vi "Launch SM DI Threads.vi"(8 "error in (no error)":errorcluster, 10 "DAQ Process AppData":T1, 11 "DAQ in":refnum<class "DAQ.lvclass">) -> (0 "error out":errorcluster, 3 "DAQ out":refnum<class "DAQ.lvclass">)   [LabVIEW 2017, in "DAQ.lvclass"]
doc: "Developed by Kevin Thompson\nkevin@thompsonengineering.net\n\nCopyright 2018-2020\nThompson Engineering, LLC"
uses:
  DAQ.lvclass
  Process_DAQ SM AppData--cluster.ctl
  DataTypes/TD DAQ Settings--cluster.ctl
  DataTypes/TD DI Instrument Settings--cluster.ctl
  DataTypes/TD AI Instrument Settings--cluster.ctl
  DataTypes/TD AI InstSettings--cluster.ctl
  TD SimAI Ranges--cluster.ctl
  <vilib>/TELLC/Dynamic CVT API/TD Dynamic CVT DVR--ref.ctl
  DAQ.lvclass/DAQ.ctl
  Accessors/Get DI TaskNames.vi
  SM_DI-DAQInstrument.vi
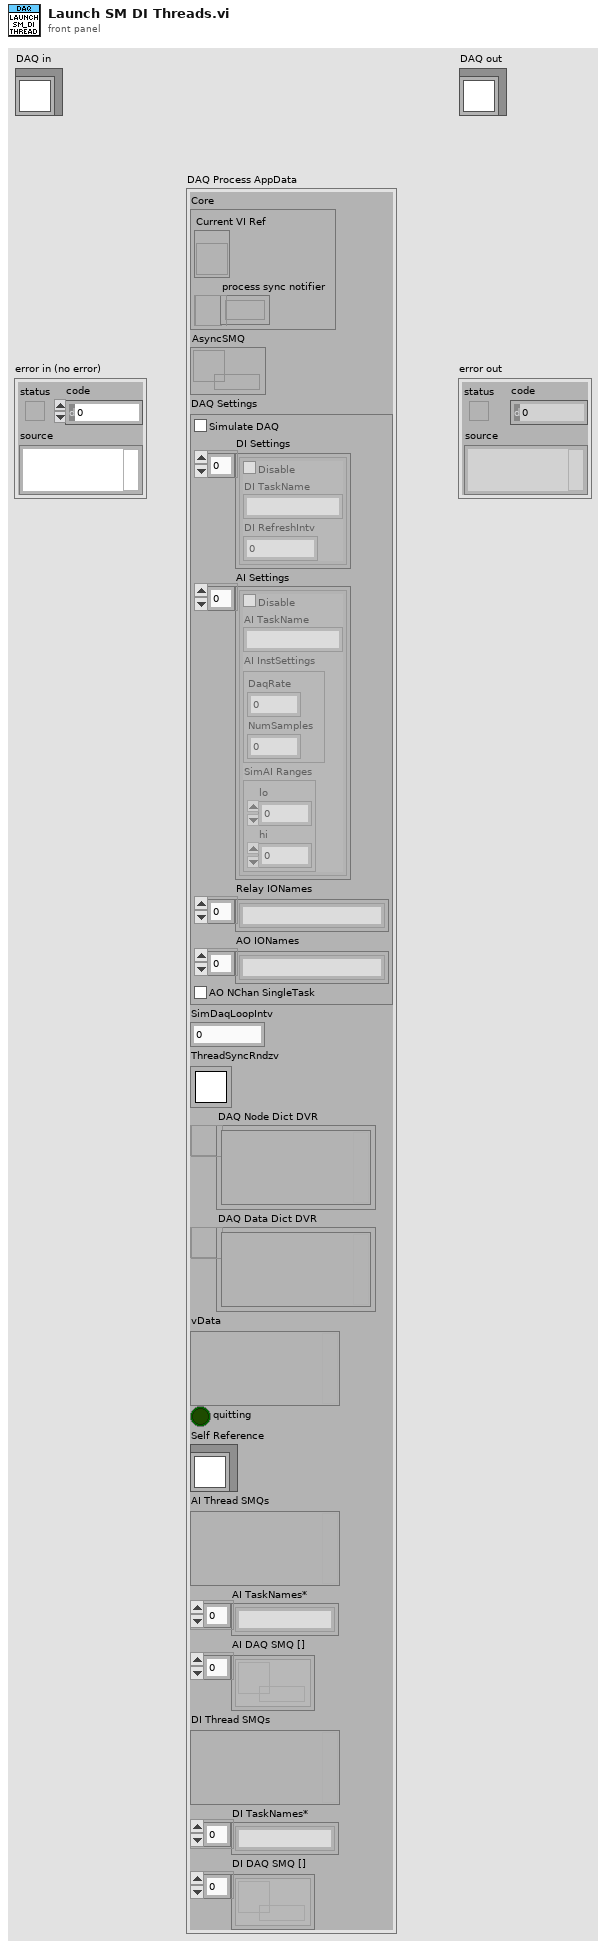
[diagram p1: front panel]
types:
  T1 = typedef "DAQ.lvclass/Process_DAQ SM AppData--cluster.ctl" = cluster{"Core":cluster{"Current VI Ref":refnum<vi>, "process sync notifier":refnum<notifier>}, "AsyncSMQ":refnum<queue>, "DAQ Settings":T2, "SimDaqLoopIntv":i32, "ThreadSyncRndzv":T7, "DAQ Node Dict DVR":T8, "DAQ Data Dict DVR":T8, "vData":variant, "quitting":bool, "Self Reference":refnum<class "DAQ.lvclass">, "AI Thread SMQs":variant, "AI TaskNames*":string[], "AI DAQ SMQ []":refnum<queue>[], "DI Thread SMQs":variant, "DI TaskNames*":string[], "DI DAQ SMQ []":refnum<queue>[]}
  T2 = typedef "DAQ.lvclass/TD DAQ Settings--cluster.ctl" = cluster{"Simulate DAQ":bool, "DI Settings":T3[], "AI Settings":T4[], "Relay IONames":string[], "AO IONames":string[], "AO NChan SingleTask":bool}
  T3 = typedef "DAQ.lvclass/TD DI Instrument Settings--cluster.ctl" = cluster{"Disable":bool, "DI TaskName":string, "DI RefreshIntv":i32}
  T4 = typedef "DAQ.lvclass/TD AI Instrument Settings--cluster.ctl" = cluster{"Disable":bool, "AI TaskName":string, "AI InstSettings":T5, "SimAI Ranges":T6}
  T5 = typedef "DAQ.lvclass/TD AI InstSettings--cluster.ctl" = cluster{"DaqRate":dbl, "NumSamples":i32}
  T6 = typedef "DAQ.lvclass/TD SimAI Ranges--cluster.ctl" = cluster{"lo":dbl, "hi":dbl}
  T7 = typedef "Rendezvous RefNum" = refnum<k1>
  T8 = typedef "TD Dynamic CVT DVR--ref.ctl" = refnum<data-value>
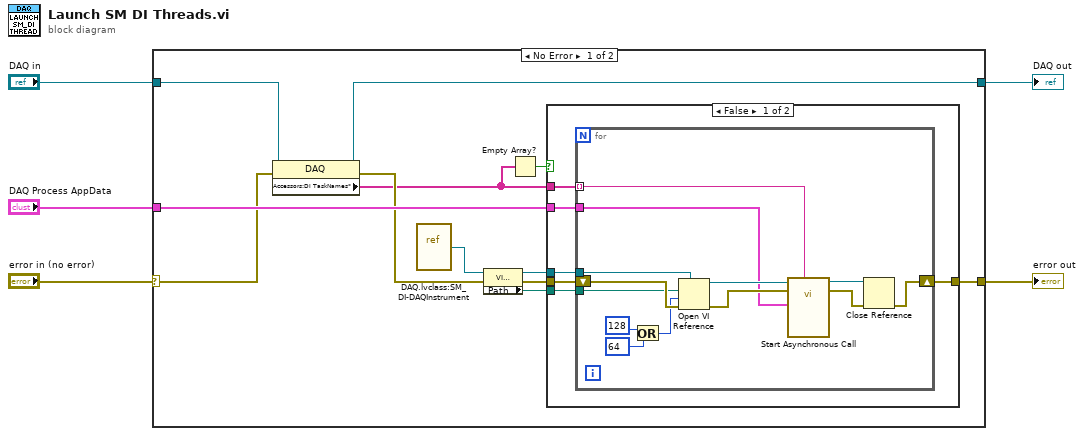
[diagram p0: block diagram]
diagram:
  n1 = case shown="No Error" "error in (no error)" {
    selector: "error in (no error)" -> [w14 w39]
    tunnel: [w13 w39] -> w4
    tunnel: [w11 w38] -> w2
    tunnel: "DAQ in" -> [w10 w38]
    tunnel: "DAQ Process AppData" -> [w15 _]
    frame No Error {
      n2 = property class="DAQ"(reference=w10, error in=w14) -> (reference out=w11:refnum<class "DAQ.lvclass">, error out=w12:errorcluster, "Accessors:DI TaskNames*"=w7:string[])
      n3 = vi-ref "DAQ.lvclass:SM_DI-DAQInstrument.vi"() -> (w9:refnum<vi>)
      n4 = property class="VI (strict)"(reference=w9, error in=w12) -> (reference out=w6:refnum<vi>, error out=w17:errorcluster, "Path"=w16:path)
      n5 = Empty Array?(array=w7) -> (empty?=w8:bool)
      n6 = case shown="False" w8 {
        tunnel: w17 -> [w23 w37]
        tunnel: w16 -> [w22 _]
        tunnel: w15 -> [w21 _]
        tunnel: w7 -> [w20 _]
        tunnel: [w19 w37] -> w13
        tunnel: w6 -> [w18 _]
        frame False {
          n7 = for {
            tunnel: w22 -> [w34]
            shift-right: [w29] -> w19
            shift-left: w23 -> [w35]
            tunnel: w21 -> [w26]
            tunnel: w20 -> [w25] mode=indexing
            tunnel: w18 -> [w24]
            n8 = Or(x=128 ("options"), y=64 ("options")) -> (x .or. y?=w31:i32)
            n9 = Open VI Reference(type specifier VI Refnum (for type only)=w24, vi path=w34, options=w31, error in (no error)=w35) -> (vi reference=w27:refnum<vi>, error out=w28:errorcluster)  [unwired: 2 in]
            n10 = call-by-ref "Start Asynchronous Call"(reference=w27, error in=w28, "DI TaskName"=w25, "DAQ Process AppData"=w26) -> (reference out=w36:refnum<vi>, error out=w30:errorcluster)  [unwired: 9 in, 1 out]
            n11 = Close Reference(reference=w36, error in (no error)=w30) -> (error out=w29:errorcluster)
          }
        }
        frame True {
        }
      }
    }
    frame Error {
    }
  }
  "error out" <- w4
  "DAQ out" <- w2
